vi "Get Daemon Status.vi"(8 "error in (no error)":errorcluster, 11 "Modbus slave in":refnum<class "Modbus Slave.lvclass">) -> (0 "error out":errorcluster, 2 "daemon status":T1, 3 "Modbus Slave out":refnum<class "Modbus Slave.lvclass">)   [LabVIEW 2012, in "Modbus Slave.lvclass"]
doc: "This VI is an accessor for the <B>daemon status</B> stored in the Modbus slave instance. This accessor can be used as a property node. This status indicates the state of the Modbus daemon."
uses:
  Modbus Slave.lvclass
  Network Protocol/Network Slave/daemon status.ctl
  Modbus Slave.lvclass/Modbus Slave.ctl
  Network Protocol/Network Slave/Network Slave.lvclass
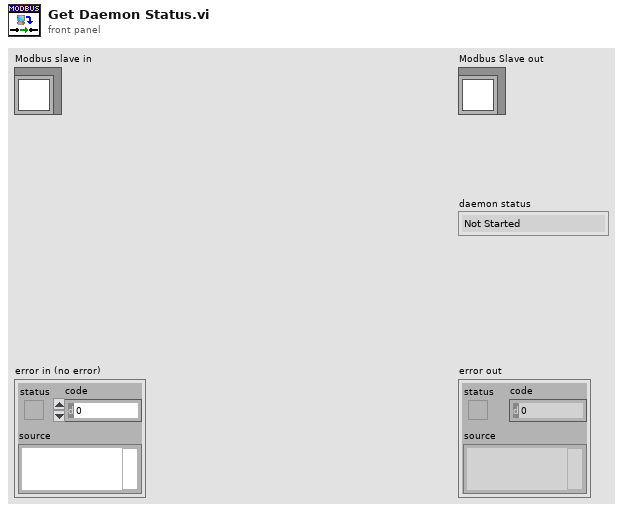
[diagram p1: front panel]
types:
  T1 = typedef "Network Slave.lvclass/daemon status.ctl" = enum16{"Not Started", "Running", "Error", "Stopped"}
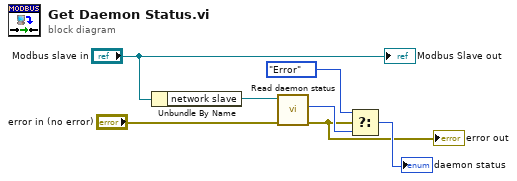
[diagram p0: block diagram]
diagram:
  n1 = Unbundle By Name("Modbus slave in") -> ("network slave"=w4:refnum<class "Network Slave.lvclass">)
  n2 = call "Read daemon status.vi"("error in (no error)"="error in (no error)", "Network Slave in"=w4) -> ("error out"=w1:errorcluster, "daemon status"=w2:T1)  [unwired: 7 in, 1 out]
  "error out" <- w1
  n3 = Select(t=daemon_status."Error", s=w1, f=w2) -> (s? t:f=→"daemon status":T1)
  "Modbus Slave out" <- "Modbus slave in"
